vi "Initialise Status Monitor Connection.vi"(8 "error in":errorcluster, 10 "timeout (ms)":i32, 11 "Address":string) -> (0 "error out":errorcluster, 3 "Status Connection Out":T1={"Description"="", "Address"="", "Port"=0, "timeout (ms)"=5000, "Termination Character"="\n", "TCP Connection Reference"=refnum, "Open Connection"=FALSE})   [LabVIEW 2017, in "Status Monitor Library.lvlib"]
doc: "Initialises and opens a connection to the status port (2234)"
uses:
  Status Monitor Library.lvlib
  Communications/Typedefs/DTACQ Connection Data--Cluster.ctl
  Communications/Communications Library.lvlib
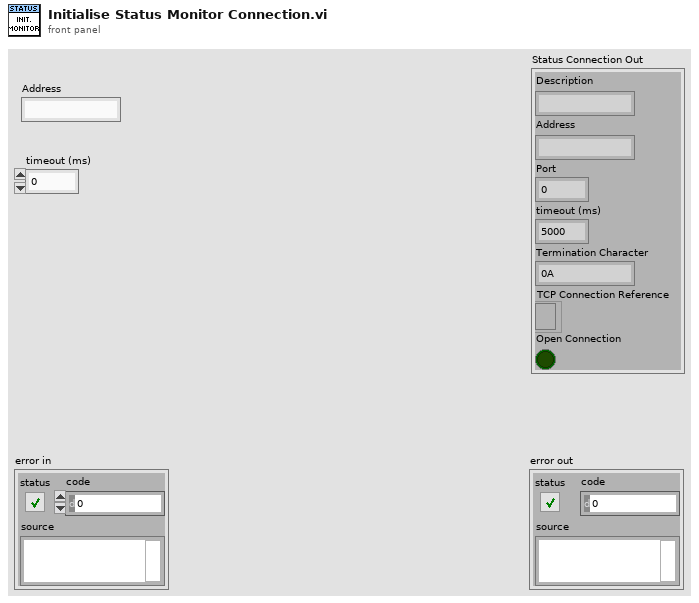
[diagram p1: front panel]
types:
  T1 = typedef "Communications Library.lvlib/DTACQ Connection Data--Cluster.ctl" = cluster{"Description":string, "Address":string, "Port":u16, "timeout (ms)":i32, "Termination Character":string, "TCP Connection Reference":refnum<k5>, "Open Connection":bool}
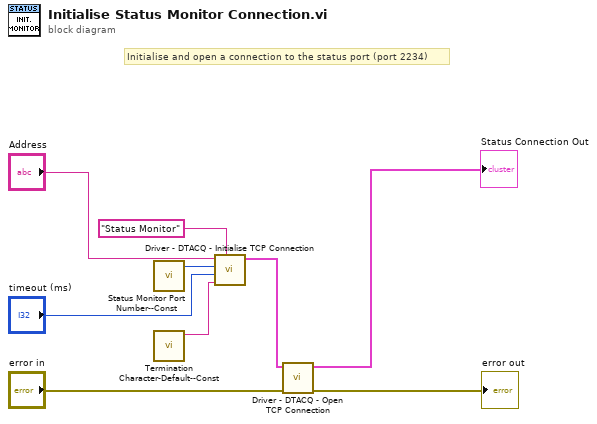
[diagram p0: block diagram]
diagram:
  # "Initialise and open a connection to the status port (port 2234)"
  n1 = call "Status Monitor Port Number--Const.vi"() -> ("Status Monitor Port"=w8:i32)  [unwired: 11 in]
  n2 = call "Termination Character-Default--Const.vi"() -> ("Termination Character"=w9:string)  [unwired: 11 in]
  n3 = call "Driver - DTACQ - Initialise TCP Connection.vi"("Description"="Status Monitor", "Termination Character"=w9, "timeout (ms)"="timeout (ms)", "Port"=w8, "Address"="Address") -> ("DTACQ Connection Data Out"=w4:T1)  [unwired: 6 in]
  n4 = call "Driver - DTACQ - Open TCP Connection.vi"("error in"="error in", "DTACQ Connection Data In"=w4) -> ("error out"=→"error out":errorcluster, "DTACQ Connection Data Out"=→"Status Connection Out":T1)  [unwired: 8 in]
